vi "Create TDMS File.vi"(8 "error in (no error)":errorcluster, 10 "LogFile Folder":path) -> (0 "error out":errorcluster, 1 "tdms ref":refnum<k34>, 2 "TDMS File Pathname":path)   [LabVIEW 2017, in "LogEngine.lvclass"]
doc: "Developed by Kevin Thompson\nkevin@thompsonengineering.net\n\nCopyright 2018-2020\nThompson Engineering, LLC"
uses:
  LogEngine.lvclass
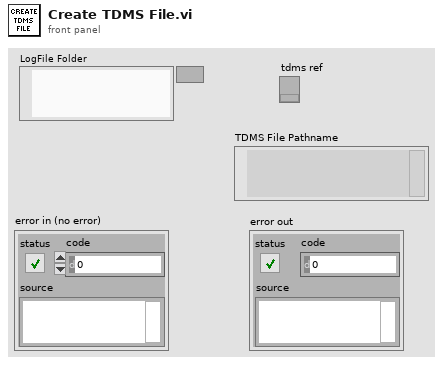
[diagram p1: front panel]
types:
  T1 = enum16{"open", "open or create", "create or replace", "create", "open (read-only)"}
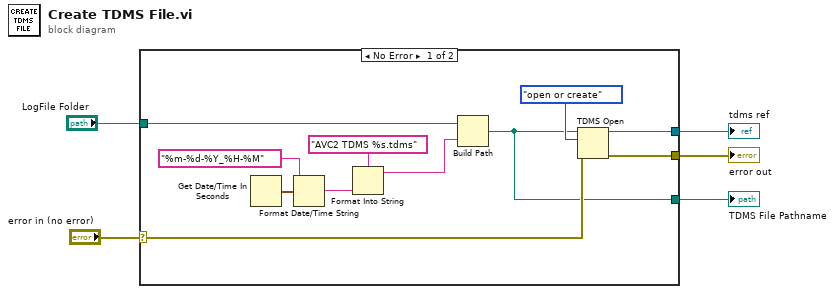
[diagram p0: block diagram]
diagram:
  n1 = case shown="No Error" "error in (no error)" {
    selector: "error in (no error)" -> [w7 w17]
    tunnel: "LogFile Folder" -> [w11 _]
    tunnel: [w10 _] -> w4
    tunnel: [w8 w17] -> w3
    tunnel: [w6 _] -> w1
    frame No Error {
      n2 = Get Date/Time In Seconds() -> (seconds since 1Jan1904=w13:timestamp)
      n3 = Format Date/Time String(time format string (%c)="%m-%d-%Y_%H-%M", seconds (now)=w13) -> (date/time string=w14:string)  [unwired: 1 in]
      n4 = Format Into String(format string="AVC2 TDMS %s.tdms", w14) -> (resulting string=w16:string)  [unwired: 2 in, 1 out]
      n5 = Build Path(base path=w11, name or relative path=w16) -> (appended path=w6:path)
      n6 = TDMS Open(8:w7, 10:T1."open or create" ("operation (0:open)"), 11:w6) -> (0:w8:errorcluster, 3:w10:refnum<k34>)  [unwired: 4 in]
    }
    frame Error {
    }
  }
  "error out" <- w3
  "tdms ref" <- w4
  "TDMS File Pathname" <- w1
